vi "main(Test DQMH modules).vi"() -> ()   [LabVIEW 2018, in "Application.lvlib"] (continued)
                n6985 = To Variant(anything=bool[] [FALSE, FALSE, TRUE, FALSE, FALSE, FALSE]) -> (Variant=w14928:variant)
                n6986 = Bundle By Name(cluster=w14931, "command"="MEAS.AllRelaysOFF") -> (w14927:T9)
                n6987 = Bundle By Name(cluster=w14931, "command"="MEAS.mux10-1", "data"=w14938) -> (w14926:T9)
                n6988 = Bundle By Name(cluster=w14931, "command"="MEAS.mux6_1", "data"=w14936) -> (w14925:T9)
                n6989 = Bundle By Name(cluster=w14931, "command"="MEAS.demux1-10", "data"=w14932) -> (w14924:T9)
                n6990 = Bundle By Name(cluster=w14931, "command"="MEAS.eMIC", "data"=w14928) -> (w14923:T9)
                n6991 = Build Array(w14927, w14926, w14925, w14924, w14923) -> (w14908:T9[])
                n6992 = To Variant(anything=w14913) -> (Variant=w14911:variant)
                n6993 = To Variant(anything=w14913) -> (Variant=w14910:variant)
                n6994 = Bundle By Name(cluster=w14909, "command"="WaitFor") -> (w14907:T9)
                n6995 = Bundle By Name(cluster=w14909, "command"="MEAS.DMM dual read") -> (w14920:T9)
                n6996 = Bundle By Name(cluster=w14909, "command"="MEAS.requestAC", "data"=w14911) -> (w14919:T9)
                n6997 = Bundle By Name(cluster=w14909, "command"="Apps.WaitForEvent", "data"=w14910) -> (w14914:T9)
                n6998 = Bundle By Name(cluster=w14909, "command"="Apps.UI Update 1") -> (w14915:T9)
                n6999 = Build Array (concatenate)(w14908, w14907, w14920, w14919, w14914, w14915) -> (w14912:T9[])
              }
            }
          }
          frame True {
            n7000 = Bundle By Name(cluster=T9 {"command"="", "data"=variant} ("element"), "command"="Apps.UI Update 1") -> (w14942:T9)
            n7001 = Build Array(w14942) -> (w14941:T9[])
          }
        }
        n7002 = for {
          tunnel: w14857 -> [w14952] mode=indexing
          tunnel: w14865 -> [w14953]
          tunnel: [w14949] -> w14867 mode=indexing
          n7003 = Unbundle By Name(w14952) -> ("command"=w14951:string, "data"=w14950:variant)
          n7004 = call "App enquece.vi"("command data"=w14950, "command"=w14951, "queue in"=w14953) -> ("error out"=w14949:errorcluster)  [unwired: 7 in, 1 out]
        }
        n7005 = Merge Errors(w14868, w14867) -> (w14866:errorcluster)
      }
      frame "Test DRV 52A" {
        w14957 = 52 ("DUT index(0-59)")
        n7006 = disable-structure shown="LOGGING==TRUE" {
          disable-tunnel: w14962 -> [w15045 _]
          frame condition #0 (active) {
            n7007 = Empty String/Path?(string/path=w15045) -> (empty?=w15047:bool)
            n7008 = Select(t="Quece timeout", s=w15047, f=w15045) -> (s? t:f=w15044:string)
            n7009 = call "string log (SubVI).vi"("state Name"=w15044) -> ()  [unwired: 9 in, 2 out]
          }
          frame condition #1 {
          }
        }
        n7010 = Flush Queue(queue=w14963) -> (queue out=w14964:refnum<queue>)  [unwired: 1 in, 2 out]
        n7011 = Decrement(x=w14957) -> (x-1=w14961:i32)
        n7012 = Index Array(array=w14958, index=w14961) -> (element=w14959:refnum<vi>)
        n7013 = call "FGV DRV stand.vi"() -> ("Sub-Test.DCV"=w14954:bool)  [unwired: 10 in, 1 out]
        n7014 = call "FGV Driver Data.vi"("DUT index(1-60)"=w14957) -> ("DUT SC"=w14955:bool)  [unwired: 7 in, 3 out]
        n7015 = property class="ColBox"(reference=w14959, "Value"=u32 10000536 ("DRV 1")) -> ()  [unwired: 1 in, 2 out]
        n7016 = case shown="False" w14955 {
          tunnel: w14957 -> [w14975 _]
          tunnel: [w14974 w15040] -> w14956
          tunnel: w14954 -> [w14973 _]
          frame False {
            n7017 = case shown="False" w14973 {
              tunnel: w14975 -> [w14982 w15012]
              tunnel: [w14993 w15011] -> w14974
              frame False {
                w14979 = T9 {"command"="", "data"=variant} ("element")
                w14992 = T9 {"command"="", "data"=variant} ("element")
                n7018 = To Variant(anything=T3."mux10_1_channel9" ("mux10_1(x6)_encode")) -> (Variant=w14990:variant)
                n7019 = To Variant(anything=T4."demux1_10_channel9" ("demux1_10(x6)_encode")) -> (Variant=w14986:variant)
                n7020 = To Variant(anything=bool[] [FALSE, FALSE, FALSE, TRUE, FALSE, FALSE]) -> (Variant=w15001:variant)
                n7021 = Bundle By Name(cluster=w14992, "command"="MEAS.AllRelaysOFF") -> (w15000:T9)
                n7022 = Bundle By Name(cluster=w14992, "command"="MEAS.mux10-1", "data"=w14990) -> (w14983:T9)
                n7023 = Bundle By Name(cluster=w14992, "command"="MEAS.demux1-10", "data"=w14986) -> (w14984:T9)
                n7024 = Bundle By Name(cluster=w14992, "command"="MEAS.eMIC", "data"=w15001) -> (w14985:T9)
                n7025 = Build Array(w15000, w14983, w14984, w14985) -> (w14978:T9[])
                n7026 = To Variant(anything=w14982) -> (Variant=w14981:variant)
                n7027 = To Variant(anything=w14982) -> (Variant=w14980:variant)
                n7028 = Bundle By Name(cluster=w14979, "command"="MEAS.requestAC", "data"=w14981) -> (w14998:T9)
                n7029 = Bundle By Name(cluster=w14979, "command"="Apps.WaitForEvent", "data"=w14980) -> (w14994:T9)
                n7030 = Bundle By Name(cluster=w14979, "command"="Apps.UI Update 1") -> (w14995:T9)
                n7031 = Bundle By Name(cluster=w14979, "command"="WaitFor") -> (w14977:T9)
                n7032 = Build Array (concatenate)(w14978, w14977, w14998, w14994, w14995) -> (w14993:T9[])
              }
              frame True {
                w15008 = T9 {"command"="", "data"=variant} ("element")
                w15030 = T9 {"command"="", "data"=variant} ("element")
                n7033 = To Variant(anything=T3."mux10_1_channel9" ("mux10_1(x6)_encode")) -> (Variant=w15037:variant)
                n7034 = To Variant(anything=T2."mux6_1_channel4_3" ("mux6_1(3wires)_encode")) -> (Variant=w15035:variant)
                n7035 = To Variant(anything=T4."demux1_10_channel9" ("demux1_10(x6)_encode")) -> (Variant=w15031:variant)
                n7036 = To Variant(anything=bool[] [FALSE, FALSE, FALSE, TRUE, FALSE, FALSE]) -> (Variant=w15027:variant)
                n7037 = Bundle By Name(cluster=w15030, "command"="MEAS.AllRelaysOFF") -> (w15026:T9)
                n7038 = Bundle By Name(cluster=w15030, "command"="MEAS.mux10-1", "data"=w15037) -> (w15025:T9)
                n7039 = Bundle By Name(cluster=w15030, "command"="MEAS.mux6_1", "data"=w15035) -> (w15024:T9)
                n7040 = Bundle By Name(cluster=w15030, "command"="MEAS.demux1-10", "data"=w15031) -> (w15023:T9)
                n7041 = Bundle By Name(cluster=w15030, "command"="MEAS.eMIC", "data"=w15027) -> (w15022:T9)
                n7042 = Build Array(w15026, w15025, w15024, w15023, w15022) -> (w15007:T9[])
                n7043 = To Variant(anything=w15012) -> (Variant=w15010:variant)
                n7044 = To Variant(anything=w15012) -> (Variant=w15009:variant)
                n7045 = Bundle By Name(cluster=w15008, "command"="WaitFor") -> (w15006:T9)
                n7046 = Bundle By Name(cluster=w15008, "command"="MEAS.DMM dual read") -> (w15019:T9)
                n7047 = Bundle By Name(cluster=w15008, "command"="MEAS.requestAC", "data"=w15010) -> (w15018:T9)
                n7048 = Bundle By Name(cluster=w15008, "command"="Apps.WaitForEvent", "data"=w15009) -> (w15013:T9)
                n7049 = Bundle By Name(cluster=w15008, "command"="Apps.UI Update 1") -> (w15014:T9)
                n7050 = Build Array (concatenate)(w15007, w15006, w15019, w15018, w15013, w15014) -> (w15011:T9[])
              }
            }
          }
          frame True {
            n7051 = Bundle By Name(cluster=T9 {"command"="", "data"=variant} ("element"), "command"="Apps.UI Update 1") -> (w15041:T9)
            n7052 = Build Array(w15041) -> (w15040:T9[])
          }
        }
        n7053 = for {
          tunnel: w14956 -> [w15051] mode=indexing
          tunnel: w14964 -> [w15052]
          tunnel: [w15048] -> w14966 mode=indexing
          n7054 = Unbundle By Name(w15051) -> ("command"=w15050:string, "data"=w15049:variant)
          n7055 = call "App enquece.vi"("command data"=w15049, "command"=w15050, "queue in"=w15052) -> ("error out"=w15048:errorcluster)  [unwired: 7 in, 1 out]
        }
        n7056 = Merge Errors(w14967, w14966) -> (w14965:errorcluster)
      }
      frame "Test DRV 53A" {
        w15056 = 53 ("DUT index(0-59)")
        n7057 = disable-structure shown="LOGGING==TRUE" {
          disable-tunnel: w15061 -> [w15144 _]
          frame condition #0 (active) {
            n7058 = Empty String/Path?(string/path=w15144) -> (empty?=w15146:bool)
            n7059 = Select(t="Quece timeout", s=w15146, f=w15144) -> (s? t:f=w15143:string)
            n7060 = call "string log (SubVI).vi"("state Name"=w15143) -> ()  [unwired: 9 in, 2 out]
          }
          frame condition #1 {
          }
        }
        n7061 = Flush Queue(queue=w15062) -> (queue out=w15063:refnum<queue>)  [unwired: 1 in, 2 out]
        n7062 = Decrement(x=w15056) -> (x-1=w15060:i32)
        n7063 = Index Array(array=w15057, index=w15060) -> (element=w15058:refnum<vi>)
        n7064 = call "FGV DRV stand.vi"() -> ("Sub-Test.DCV"=w15053:bool)  [unwired: 10 in, 1 out]
        n7065 = call "FGV Driver Data.vi"("DUT index(1-60)"=w15056) -> ("DUT SC"=w15054:bool)  [unwired: 7 in, 3 out]
        n7066 = property class="ColBox"(reference=w15058, "Value"=u32 10000536 ("DRV 1")) -> ()  [unwired: 1 in, 2 out]
        n7067 = case shown="False" w15054 {
          tunnel: w15056 -> [w15074 _]
          tunnel: [w15073 w15139] -> w15055
          tunnel: w15053 -> [w15072 _]
          frame False {
            n7068 = case shown="True" w15072 {
              tunnel: w15074 -> [w15081 w15111]
              tunnel: [w15092 w15110] -> w15073
              frame False {
                w15078 = T9 {"command"="", "data"=variant} ("element")
                w15091 = T9 {"command"="", "data"=variant} ("element")
                n7069 = To Variant(anything=T3."mux10_1_channel9" ("mux10_1(x6)_encode")) -> (Variant=w15089:variant)
                n7070 = To Variant(anything=T4."demux1_10_channel9" ("demux1_10(x6)_encode")) -> (Variant=w15085:variant)
                n7071 = To Variant(anything=bool[] [FALSE, FALSE, FALSE, FALSE, TRUE, FALSE]) -> (Variant=w15100:variant)
                n7072 = Bundle By Name(cluster=w15091, "command"="MEAS.AllRelaysOFF") -> (w15099:T9)
                n7073 = Bundle By Name(cluster=w15091, "command"="MEAS.mux10-1", "data"=w15089) -> (w15082:T9)
                n7074 = Bundle By Name(cluster=w15091, "command"="MEAS.demux1-10", "data"=w15085) -> (w15083:T9)
                n7075 = Bundle By Name(cluster=w15091, "command"="MEAS.eMIC", "data"=w15100) -> (w15084:T9)
                n7076 = Build Array(w15099, w15082, w15083, w15084) -> (w15077:T9[])
                n7077 = To Variant(anything=w15081) -> (Variant=w15080:variant)
                n7078 = To Variant(anything=w15081) -> (Variant=w15079:variant)
                n7079 = Bundle By Name(cluster=w15078, "command"="MEAS.requestAC", "data"=w15080) -> (w15097:T9)
                n7080 = Bundle By Name(cluster=w15078, "command"="Apps.WaitForEvent", "data"=w15079) -> (w15093:T9)
                n7081 = Bundle By Name(cluster=w15078, "command"="Apps.UI Update 1") -> (w15094:T9)
                n7082 = Bundle By Name(cluster=w15078, "command"="WaitFor") -> (w15076:T9)
                n7083 = Build Array (concatenate)(w15077, w15076, w15097, w15093, w15094) -> (w15092:T9[])
              }
              frame True {
                w15107 = T9 {"command"="", "data"=variant} ("element")
                w15129 = T9 {"command"="", "data"=variant} ("element")
                n7084 = To Variant(anything=T3."mux10_1_channel9" ("mux10_1(x6)_encode")) -> (Variant=w15136:variant)
                n7085 = To Variant(anything=T2."mux6_1_channel5_3" ("mux6_1(3wires)_encode")) -> (Variant=w15134:variant)
                n7086 = To Variant(anything=T4."demux1_10_channel9" ("demux1_10(x6)_encode")) -> (Variant=w15130:variant)
                n7087 = To Variant(anything=bool[] [FALSE, FALSE, FALSE, FALSE, TRUE, FALSE]) -> (Variant=w15126:variant)
                n7088 = Bundle By Name(cluster=w15129, "command"="MEAS.AllRelaysOFF") -> (w15125:T9)
                n7089 = Bundle By Name(cluster=w15129, "command"="MEAS.mux10-1", "data"=w15136) -> (w15124:T9)
                n7090 = Bundle By Name(cluster=w15129, "command"="MEAS.mux6_1", "data"=w15134) -> (w15123:T9)
                n7091 = Bundle By Name(cluster=w15129, "command"="MEAS.demux1-10", "data"=w15130) -> (w15122:T9)
                n7092 = Bundle By Name(cluster=w15129, "command"="MEAS.eMIC", "data"=w15126) -> (w15121:T9)
                n7093 = Build Array(w15125, w15124, w15123, w15122, w15121) -> (w15106:T9[])
                n7094 = To Variant(anything=w15111) -> (Variant=w15109:variant)
                n7095 = To Variant(anything=w15111) -> (Variant=w15108:variant)
                n7096 = Bundle By Name(cluster=w15107, "command"="WaitFor") -> (w15105:T9)
                n7097 = Bundle By Name(cluster=w15107, "command"="MEAS.DMM dual read") -> (w15118:T9)
                n7098 = Bundle By Name(cluster=w15107, "command"="MEAS.requestAC", "data"=w15109) -> (w15117:T9)
                n7099 = Bundle By Name(cluster=w15107, "command"="Apps.WaitForEvent", "data"=w15108) -> (w15112:T9)
                n7100 = Bundle By Name(cluster=w15107, "command"="Apps.UI Update 1") -> (w15113:T9)
                n7101 = Build Array (concatenate)(w15106, w15105, w15118, w15117, w15112, w15113) -> (w15110:T9[])
              }
            }
          }
          frame True {
            n7102 = Bundle By Name(cluster=T9 {"command"="", "data"=variant} ("element"), "command"="Apps.UI Update 1") -> (w15140:T9)
            n7103 = Build Array(w15140) -> (w15139:T9[])
          }
        }
        n7104 = for {
          tunnel: w15055 -> [w15150] mode=indexing
          tunnel: w15063 -> [w15151]
          tunnel: [w15147] -> w15065 mode=indexing
          n7105 = Unbundle By Name(w15150) -> ("command"=w15149:string, "data"=w15148:variant)
          n7106 = call "App enquece.vi"("command data"=w15148, "command"=w15149, "queue in"=w15151) -> ("error out"=w15147:errorcluster)  [unwired: 7 in, 1 out]
        }
        n7107 = Merge Errors(w15066, w15065) -> (w15064:errorcluster)
      }
      frame "Test DRV 54A" {
        w15155 = 54 ("DUT index(0-59)")
        n7108 = disable-structure shown="LOGGING==TRUE" {
          disable-tunnel: w15160 -> [w15243 _]
          frame condition #0 (active) {
            n7109 = Empty String/Path?(string/path=w15243) -> (empty?=w15245:bool)
            n7110 = Select(t="Quece timeout", s=w15245, f=w15243) -> (s? t:f=w15242:string)
            n7111 = call "string log (SubVI).vi"("state Name"=w15242) -> ()  [unwired: 9 in, 2 out]
          }
          frame condition #1 {
          }
        }
        n7112 = Flush Queue(queue=w15161) -> (queue out=w15162:refnum<queue>)  [unwired: 1 in, 2 out]
        n7113 = Decrement(x=w15155) -> (x-1=w15159:i32)
        n7114 = Index Array(array=w15156, index=w15159) -> (element=w15157:refnum<vi>)
        n7115 = call "FGV DRV stand.vi"() -> ("Sub-Test.DCV"=w15152:bool)  [unwired: 10 in, 1 out]
        n7116 = call "FGV Driver Data.vi"("DUT index(1-60)"=w15155) -> ("DUT SC"=w15153:bool)  [unwired: 7 in, 3 out]
        n7117 = property class="ColBox"(reference=w15157, "Value"=u32 10000536 ("DRV 1")) -> ()  [unwired: 1 in, 2 out]
        n7118 = case shown="False" w15153 {
          tunnel: w15155 -> [w15173 _]
          tunnel: [w15172 w15238] -> w15154
          tunnel: w15152 -> [w15171 _]
          frame False {
            n7119 = case shown="False" w15171 {
              tunnel: w15173 -> [w15180 w15210]
              tunnel: [w15191 w15209] -> w15172
              frame False {
                w15177 = T9 {"command"="", "data"=variant} ("element")
                w15190 = T9 {"command"="", "data"=variant} ("element")
                n7120 = To Variant(anything=T3."mux10_1_channel9" ("mux10_1(x6)_encode")) -> (Variant=w15188:variant)
                n7121 = To Variant(anything=T4."demux1_10_channel9" ("demux1_10(x6)_encode")) -> (Variant=w15184:variant)
                n7122 = To Variant(anything=bool[] [FALSE, FALSE, FALSE, FALSE, FALSE, TRUE]) -> (Variant=w15199:variant)
                n7123 = Bundle By Name(cluster=w15190, "command"="MEAS.AllRelaysOFF") -> (w15198:T9)
                n7124 = Bundle By Name(cluster=w15190, "command"="MEAS.mux10-1", "data"=w15188) -> (w15181:T9)
                n7125 = Bundle By Name(cluster=w15190, "command"="MEAS.demux1-10", "data"=w15184) -> (w15182:T9)
                n7126 = Bundle By Name(cluster=w15190, "command"="MEAS.eMIC", "data"=w15199) -> (w15183:T9)
                n7127 = Build Array(w15198, w15181, w15182, w15183) -> (w15176:T9[])
                n7128 = To Variant(anything=w15180) -> (Variant=w15179:variant)
                n7129 = To Variant(anything=w15180) -> (Variant=w15178:variant)
                n7130 = Bundle By Name(cluster=w15177, "command"="MEAS.requestAC", "data"=w15179) -> (w15196:T9)
                n7131 = Bundle By Name(cluster=w15177, "command"="Apps.WaitForEvent", "data"=w15178) -> (w15192:T9)
                n7132 = Bundle By Name(cluster=w15177, "command"="Apps.UI Update 1") -> (w15193:T9)
                n7133 = Bundle By Name(cluster=w15177, "command"="WaitFor") -> (w15175:T9)
                n7134 = Build Array (concatenate)(w15176, w15175, w15196, w15192, w15193) -> (w15191:T9[])
              }
              frame True {
                w15206 = T9 {"command"="", "data"=variant} ("element")
                w15228 = T9 {"command"="", "data"=variant} ("element")
                n7135 = To Variant(anything=T3."mux10_1_channel9" ("mux10_1(x6)_encode")) -> (Variant=w15235:variant)
                n7136 = To Variant(anything=T2."mux6_1_channel6_3" ("mux6_1(3wires)_encode")) -> (Variant=w15233:variant)
                n7137 = To Variant(anything=T4."demux1_10_channel9" ("demux1_10(x6)_encode")) -> (Variant=w15229:variant)
                n7138 = To Variant(anything=bool[] [FALSE, FALSE, FALSE, FALSE, FALSE, TRUE]) -> (Variant=w15225:variant)
                n7139 = Bundle By Name(cluster=w15228, "command"="MEAS.AllRelaysOFF") -> (w15224:T9)
                n7140 = Bundle By Name(cluster=w15228, "command"="MEAS.mux10-1", "data"=w15235) -> (w15223:T9)
                n7141 = Bundle By Name(cluster=w15228, "command"="MEAS.mux6_1", "data"=w15233) -> (w15222:T9)
                n7142 = Bundle By Name(cluster=w15228, "command"="MEAS.demux1-10", "data"=w15229) -> (w15221:T9)
                n7143 = Bundle By Name(cluster=w15228, "command"="MEAS.eMIC", "data"=w15225) -> (w15220:T9)
                n7144 = Build Array(w15224, w15223, w15222, w15221, w15220) -> (w15205:T9[])
                n7145 = To Variant(anything=w15210) -> (Variant=w15208:variant)
                n7146 = To Variant(anything=w15210) -> (Variant=w15207:variant)
                n7147 = Bundle By Name(cluster=w15206, "command"="WaitFor") -> (w15204:T9)
                n7148 = Bundle By Name(cluster=w15206, "command"="MEAS.DMM dual read") -> (w15217:T9)
                n7149 = Bundle By Name(cluster=w15206, "command"="MEAS.requestAC", "data"=w15208) -> (w15216:T9)
                n7150 = Bundle By Name(cluster=w15206, "command"="Apps.WaitForEvent", "data"=w15207) -> (w15211:T9)
                n7151 = Bundle By Name(cluster=w15206, "command"="Apps.UI Update 1") -> (w15212:T9)
                n7152 = Build Array (concatenate)(w15205, w15204, w15217, w15216, w15211, w15212) -> (w15209:T9[])
              }
            }
          }
          frame True {
            n7153 = Bundle By Name(cluster=T9 {"command"="", "data"=variant} ("element"), "command"="Apps.UI Update 1") -> (w15239:T9)
            n7154 = Build Array(w15239) -> (w15238:T9[])
          }
        }
        n7155 = for {
          tunnel: w15154 -> [w15249] mode=indexing
          tunnel: w15162 -> [w15250]
          tunnel: [w15246] -> w15164 mode=indexing
          n7156 = Unbundle By Name(w15249) -> ("command"=w15248:string, "data"=w15247:variant)
          n7157 = call "App enquece.vi"("command data"=w15247, "command"=w15248, "queue in"=w15250) -> ("error out"=w15246:errorcluster)  [unwired: 7 in, 1 out]
        }
        n7158 = Merge Errors(w15165, w15164) -> (w15163:errorcluster)
      }
      frame "Test DRV 55A" {
        w15254 = 55 ("DUT index(0-59)")
        n7159 = disable-structure shown="LOGGING==TRUE" {
          disable-tunnel: w15259 -> [w15342 _]
          frame condition #0 (active) {
            n7160 = Empty String/Path?(string/path=w15342) -> (empty?=w15344:bool)
            n7161 = Select(t="Quece timeout", s=w15344, f=w15342) -> (s? t:f=w15341:string)
            n7162 = call "string log (SubVI).vi"("state Name"=w15341) -> ()  [unwired: 9 in, 2 out]
          }
          frame condition #1 {
          }
        }
        n7163 = Flush Queue(queue=w15260) -> (queue out=w15261:refnum<queue>)  [unwired: 1 in, 2 out]
        n7164 = Decrement(x=w15254) -> (x-1=w15258:i32)
        n7165 = Index Array(array=w15255, index=w15258) -> (element=w15256:refnum<vi>)
        n7166 = call "FGV DRV stand.vi"() -> ("Sub-Test.DCV"=w15251:bool)  [unwired: 10 in, 1 out]
        n7167 = call "FGV Driver Data.vi"("DUT index(1-60)"=w15254) -> ("DUT SC"=w15252:bool)  [unwired: 7 in, 3 out]
        n7168 = property class="ColBox"(reference=w15256, "Value"=u32 10000536 ("DRV 1")) -> ()  [unwired: 1 in, 2 out]
        n7169 = case shown="False" w15252 {
          tunnel: w15254 -> [w15272 _]
          tunnel: [w15271 w15337] -> w15253
          tunnel: w15251 -> [w15270 _]
          frame False {
            n7170 = case shown="True" w15270 {
              tunnel: w15272 -> [w15279 w15309]
              tunnel: [w15290 w15308] -> w15271
              frame False {
                w15276 = T9 {"command"="", "data"=variant} ("element")
                w15289 = T9 {"command"="", "data"=variant} ("element")
                n7171 = To Variant(anything=T3."mux10_1_channel10" ("mux10_1(x6)_encode")) -> (Variant=w15287:variant)
                n7172 = To Variant(anything=T4."demux1_10_channel10" ("demux1_10(x6)_encode")) -> (Variant=w15283:variant)
                n7173 = To Variant(anything=bool[] [TRUE, FALSE, FALSE, FALSE, FALSE, FALSE]) -> (Variant=w15298:variant)
                n7174 = Bundle By Name(cluster=w15289, "command"="MEAS.AllRelaysOFF") -> (w15297:T9)
                n7175 = Bundle By Name(cluster=w15289, "command"="MEAS.mux10-1", "data"=w15287) -> (w15280:T9)
                n7176 = Bundle By Name(cluster=w15289, "command"="MEAS.demux1-10", "data"=w15283) -> (w15281:T9)
                n7177 = Bundle By Name(cluster=w15289, "command"="MEAS.eMIC", "data"=w15298) -> (w15282:T9)
                n7178 = Build Array(w15297, w15280, w15281, w15282) -> (w15275:T9[])
                n7179 = To Variant(anything=w15279) -> (Variant=w15278:variant)
                n7180 = To Variant(anything=w15279) -> (Variant=w15277:variant)
                n7181 = Bundle By Name(cluster=w15276, "command"="MEAS.requestAC", "data"=w15278) -> (w15295:T9)
                n7182 = Bundle By Name(cluster=w15276, "command"="Apps.WaitForEvent", "data"=w15277) -> (w15291:T9)
                n7183 = Bundle By Name(cluster=w15276, "command"="Apps.UI Update 1") -> (w15292:T9)
                n7184 = Bundle By Name(cluster=w15276, "command"="WaitFor") -> (w15274:T9)
                n7185 = Build Array (concatenate)(w15275, w15274, w15295, w15291, w15292) -> (w15290:T9[])
              }
              frame True {
                w15305 = T9 {"command"="", "data"=variant} ("element")
                w15327 = T9 {"command"="", "data"=variant} ("element")
                n7186 = To Variant(anything=T3."mux10_1_channel10" ("mux10_1(x6)_encode")) -> (Variant=w15334:variant)
                n7187 = To Variant(anything=T2."mux6_1_channel1_3" ("mux6_1(3wires)_encode")) -> (Variant=w15332:variant)
                n7188 = To Variant(anything=T4."demux1_10_channel10" ("demux1_10(x6)_encode")) -> (Variant=w15328:variant)
                n7189 = To Variant(anything=bool[] [TRUE, FALSE, FALSE, FALSE, FALSE, FALSE]) -> (Variant=w15324:variant)
                n7190 = Bundle By Name(cluster=w15327, "command"="MEAS.AllRelaysOFF") -> (w15323:T9)
                n7191 = Bundle By Name(cluster=w15327, "command"="MEAS.mux10-1", "data"=w15334) -> (w15322:T9)
                n7192 = Bundle By Name(cluster=w15327, "command"="MEAS.mux6_1", "data"=w15332) -> (w15321:T9)
                n7193 = Bundle By Name(cluster=w15327, "command"="MEAS.demux1-10", "data"=w15328) -> (w15320:T9)
                n7194 = Bundle By Name(cluster=w15327, "command"="MEAS.eMIC", "data"=w15324) -> (w15319:T9)
                n7195 = Build Array(w15323, w15322, w15321, w15320, w15319) -> (w15304:T9[])
                n7196 = To Variant(anything=w15309) -> (Variant=w15307:variant)
                n7197 = To Variant(anything=w15309) -> (Variant=w15306:variant)
                n7198 = Bundle By Name(cluster=w15305, "command"="WaitFor") -> (w15303:T9)
                n7199 = Bundle By Name(cluster=w15305, "command"="MEAS.DMM dual read") -> (w15316:T9)
                n7200 = Bundle By Name(cluster=w15305, "command"="MEAS.requestAC", "data"=w15307) -> (w15315:T9)
                n7201 = Bundle By Name(cluster=w15305, "command"="Apps.WaitForEvent", "data"=w15306) -> (w15310:T9)
                n7202 = Bundle By Name(cluster=w15305, "command"="Apps.UI Update 1") -> (w15311:T9)
                n7203 = Build Array (concatenate)(w15304, w15303, w15316, w15315, w15310, w15311) -> (w15308:T9[])
              }
            }
          }
          frame True {
            n7204 = Bundle By Name(cluster=T9 {"command"="", "data"=variant} ("element"), "command"="Apps.UI Update 1") -> (w15338:T9)
            n7205 = Build Array(w15338) -> (w15337:T9[])
          }
        }
        n7206 = for {
          tunnel: w15253 -> [w15348] mode=indexing
          tunnel: w15261 -> [w15349]
          tunnel: [w15345] -> w15263 mode=indexing
          n7207 = Unbundle By Name(w15348) -> ("command"=w15347:string, "data"=w15346:variant)
          n7208 = call "App enquece.vi"("command data"=w15346, "command"=w15347, "queue in"=w15349) -> ("error out"=w15345:errorcluster)  [unwired: 7 in, 1 out]
        }
        n7209 = Merge Errors(w15264, w15263) -> (w15262:errorcluster)
      }
      frame "Test DRV 56A" {
        w15353 = 56 ("DUT index(0-59)")
        n7210 = disable-structure shown="LOGGING==TRUE" {
          disable-tunnel: w15358 -> [w15441 _]
          frame condition #0 (active) {
            n7211 = Empty String/Path?(string/path=w15441) -> (empty?=w15443:bool)
            n7212 = Select(t="Quece timeout", s=w15443, f=w15441) -> (s? t:f=w15440:string)
            n7213 = call "string log (SubVI).vi"("state Name"=w15440) -> ()  [unwired: 9 in, 2 out]
          }
          frame condition #1 {
          }
        }
        n7214 = Flush Queue(queue=w15359) -> (queue out=w15360:refnum<queue>)  [unwired: 1 in, 2 out]
        n7215 = Decrement(x=w15353) -> (x-1=w15357:i32)
        n7216 = Index Array(array=w15354, index=w15357) -> (element=w15355:refnum<vi>)
        n7217 = call "FGV DRV stand.vi"() -> ("Sub-Test.DCV"=w15350:bool)  [unwired: 10 in, 1 out]
        n7218 = call "FGV Driver Data.vi"("DUT index(1-60)"=w15353) -> ("DUT SC"=w15351:bool)  [unwired: 7 in, 3 out]
        n7219 = property class="ColBox"(reference=w15355, "Value"=u32 10000536 ("DRV 1")) -> ()  [unwired: 1 in, 2 out]
        n7220 = case shown="False" w15351 {
          tunnel: w15353 -> [w15371 _]
          tunnel: [w15370 w15436] -> w15352
          tunnel: w15350 -> [w15369 _]
          frame False {
            n7221 = case shown="False" w15369 {
              tunnel: w15371 -> [w15378 w15408]
              tunnel: [w15389 w15407] -> w15370
              frame False {
                w15375 = T9 {"command"="", "data"=variant} ("element")
                w15388 = T9 {"command"="", "data"=variant} ("element")
                n7222 = To Variant(anything=T3."mux10_1_channel10" ("mux10_1(x6)_encode")) -> (Variant=w15386:variant)
                n7223 = To Variant(anything=T4."demux1_10_channel10" ("demux1_10(x6)_encode")) -> (Variant=w15382:variant)
                n7224 = To Variant(anything=bool[] [FALSE, TRUE, FALSE, FALSE, FALSE, FALSE]) -> (Variant=w15397:variant)
                n7225 = Bundle By Name(cluster=w15388, "command"="MEAS.AllRelaysOFF") -> (w15396:T9)
                n7226 = Bundle By Name(cluster=w15388, "command"="MEAS.mux10-1", "data"=w15386) -> (w15379:T9)
                n7227 = Bundle By Name(cluster=w15388, "command"="MEAS.demux1-10", "data"=w15382) -> (w15380:T9)
                n7228 = Bundle By Name(cluster=w15388, "command"="MEAS.eMIC", "data"=w15397) -> (w15381:T9)
                n7229 = Build Array(w15396, w15379, w15380, w15381) -> (w15374:T9[])
                n7230 = To Variant(anything=w15378) -> (Variant=w15377:variant)
                n7231 = To Variant(anything=w15378) -> (Variant=w15376:variant)
                n7232 = Bundle By Name(cluster=w15375, "command"="MEAS.requestAC", "data"=w15377) -> (w15394:T9)
                n7233 = Bundle By Name(cluster=w15375, "command"="Apps.WaitForEvent", "data"=w15376) -> (w15390:T9)
                n7234 = Bundle By Name(cluster=w15375, "command"="Apps.UI Update 1") -> (w15391:T9)
                n7235 = Bundle By Name(cluster=w15375, "command"="WaitFor") -> (w15373:T9)
                n7236 = Build Array (concatenate)(w15374, w15373, w15394, w15390, w15391) -> (w15389:T9[])
              }
              frame True {
                w15404 = T9 {"command"="", "data"=variant} ("element")
                w15426 = T9 {"command"="", "data"=variant} ("element")
                n7237 = To Variant(anything=T3."mux10_1_channel10" ("mux10_1(x6)_encode")) -> (Variant=w15433:variant)
                n7238 = To Variant(anything=T2."mux6_1_channel2_3" ("mux6_1(3wires)_encode")) -> (Variant=w15431:variant)
                n7239 = To Variant(anything=T4."demux1_10_channel10" ("demux1_10(x6)_encode")) -> (Variant=w15427:variant)
                n7240 = To Variant(anything=bool[] [FALSE, TRUE, FALSE, FALSE, FALSE, FALSE]) -> (Variant=w15423:variant)
                n7241 = Bundle By Name(cluster=w15426, "command"="MEAS.AllRelaysOFF") -> (w15422:T9)
                n7242 = Bundle By Name(cluster=w15426, "command"="MEAS.mux10-1", "data"=w15433) -> (w15421:T9)
                n7243 = Bundle By Name(cluster=w15426, "command"="MEAS.mux6_1", "data"=w15431) -> (w15420:T9)
                n7244 = Bundle By Name(cluster=w15426, "command"="MEAS.demux1-10", "data"=w15427) -> (w15419:T9)
                n7245 = Bundle By Name(cluster=w15426, "command"="MEAS.eMIC", "data"=w15423) -> (w15418:T9)
                n7246 = Build Array(w15422, w15421, w15420, w15419, w15418) -> (w15403:T9[])
                n7247 = To Variant(anything=w15408) -> (Variant=w15406:variant)
                n7248 = To Variant(anything=w15408) -> (Variant=w15405:variant)
                n7249 = Bundle By Name(cluster=w15404, "command"="WaitFor") -> (w15402:T9)
                n7250 = Bundle By Name(cluster=w15404, "command"="MEAS.DMM dual read") -> (w15415:T9)
                n7251 = Bundle By Name(cluster=w15404, "command"="MEAS.requestAC", "data"=w15406) -> (w15414:T9)
                n7252 = Bundle By Name(cluster=w15404, "command"="Apps.WaitForEvent", "data"=w15405) -> (w15409:T9)
                n7253 = Bundle By Name(cluster=w15404, "command"="Apps.UI Update 1") -> (w15410:T9)
                n7254 = Build Array (concatenate)(w15403, w15402, w15415, w15414, w15409, w15410) -> (w15407:T9[])
              }
            }
          }
          frame True {
            n7255 = Bundle By Name(cluster=T9 {"command"="", "data"=variant} ("element"), "command"="Apps.UI Update 1") -> (w15437:T9)
            n7256 = Build Array(w15437) -> (w15436:T9[])
          }
        }
        n7257 = for {
          tunnel: w15352 -> [w15447] mode=indexing
          tunnel: w15360 -> [w15448]
          tunnel: [w15444] -> w15362 mode=indexing
          n7258 = Unbundle By Name(w15447) -> ("command"=w15446:string, "data"=w15445:variant)
          n7259 = call "App enquece.vi"("command data"=w15445, "command"=w15446, "queue in"=w15448) -> ("error out"=w15444:errorcluster)  [unwired: 7 in, 1 out]
        }
        n7260 = Merge Errors(w15363, w15362) -> (w15361:errorcluster)
      }
      frame "Test DRV 57A" {
        w15452 = 57 ("DUT index(0-59)")
        n7261 = disable-structure shown="LOGGING==TRUE" {
          disable-tunnel: w15457 -> [w15540 _]
          frame condition #0 (active) {
            n7262 = Empty String/Path?(string/path=w15540) -> (empty?=w15542:bool)
            n7263 = Select(t="Quece timeout", s=w15542, f=w15540) -> (s? t:f=w15539:string)
            n7264 = call "string log (SubVI).vi"("state Name"=w15539) -> ()  [unwired: 9 in, 2 out]
          }
          frame condition #1 {
          }
        }
        n7265 = Flush Queue(queue=w15458) -> (queue out=w15459:refnum<queue>)  [unwired: 1 in, 2 out]
        n7266 = Decrement(x=w15452) -> (x-1=w15456:i32)
        n7267 = Index Array(array=w15453, index=w15456) -> (element=w15454:refnum<vi>)
        n7268 = call "FGV DRV stand.vi"() -> ("Sub-Test.DCV"=w15449:bool)  [unwired: 10 in, 1 out]
        n7269 = call "FGV Driver Data.vi"("DUT index(1-60)"=w15452) -> ("DUT SC"=w15450:bool)  [unwired: 7 in, 3 out]
        n7270 = property class="ColBox"(reference=w15454, "Value"=u32 10000536 ("DRV 1")) -> ()  [unwired: 1 in, 2 out]
        n7271 = case shown="False" w15450 {
          tunnel: w15452 -> [w15470 _]
          tunnel: [w15469 w15535] -> w15451
          tunnel: w15449 -> [w15468 _]
          frame False {
            n7272 = case shown="True" w15468 {
              tunnel: w15470 -> [w15477 w15507]
              tunnel: [w15488 w15506] -> w15469
              frame False {
                w15474 = T9 {"command"="", "data"=variant} ("element")
                w15487 = T9 {"command"="", "data"=variant} ("element")
                n7273 = To Variant(anything=T3."mux10_1_channel10" ("mux10_1(x6)_encode")) -> (Variant=w15485:variant)
                n7274 = To Variant(anything=T4."demux1_10_channel10" ("demux1_10(x6)_encode")) -> (Variant=w15481:variant)
                n7275 = To Variant(anything=bool[] [FALSE, FALSE, TRUE, FALSE, FALSE, FALSE]) -> (Variant=w15496:variant)
                n7276 = Bundle By Name(cluster=w15487, "command"="MEAS.AllRelaysOFF") -> (w15495:T9)
                n7277 = Bundle By Name(cluster=w15487, "command"="MEAS.mux10-1", "data"=w15485) -> (w15478:T9)
                n7278 = Bundle By Name(cluster=w15487, "command"="MEAS.demux1-10", "data"=w15481) -> (w15479:T9)
                n7279 = Bundle By Name(cluster=w15487, "command"="MEAS.eMIC", "data"=w15496) -> (w15480:T9)
                n7280 = Build Array(w15495, w15478, w15479, w15480) -> (w15473:T9[])
                n7281 = To Variant(anything=w15477) -> (Variant=w15476:variant)
                n7282 = To Variant(anything=w15477) -> (Variant=w15475:variant)
                n7283 = Bundle By Name(cluster=w15474, "command"="MEAS.requestAC", "data"=w15476) -> (w15493:T9)
                n7284 = Bundle By Name(cluster=w15474, "command"="Apps.WaitForEvent", "data"=w15475) -> (w15489:T9)
                n7285 = Bundle By Name(cluster=w15474, "command"="Apps.UI Update 1") -> (w15490:T9)
                n7286 = Bundle By Name(cluster=w15474, "command"="WaitFor") -> (w15472:T9)
                n7287 = Build Array (concatenate)(w15473, w15472, w15493, w15489, w15490) -> (w15488:T9[])
              }
              frame True {
                w15503 = T9 {"command"="", "data"=variant} ("element")
                w15525 = T9 {"command"="", "data"=variant} ("element")
                n7288 = To Variant(anything=T3."mux10_1_channel10" ("mux10_1(x6)_encode")) -> (Variant=w15532:variant)
                n7289 = To Variant(anything=T2."mux6_1_channel3_3" ("mux6_1(3wires)_encode")) -> (Variant=w15530:variant)
                n7290 = To Variant(anything=T4."demux1_10_channel10" ("demux1_10(x6)_encode")) -> (Variant=w15526:variant)
                n7291 = To Variant(anything=bool[] [FALSE, FALSE, TRUE, FALSE, FALSE, FALSE]) -> (Variant=w15522:variant)
                n7292 = Bundle By Name(cluster=w15525, "command"="MEAS.AllRelaysOFF") -> (w15521:T9)
                n7293 = Bundle By Name(cluster=w15525, "command"="MEAS.mux10-1", "data"=w15532) -> (w15520:T9)
                n7294 = Bundle By Name(cluster=w15525, "command"="MEAS.mux6_1", "data"=w15530) -> (w15519:T9)
                n7295 = Bundle By Name(cluster=w15525, "command"="MEAS.demux1-10", "data"=w15526) -> (w15518:T9)
                n7296 = Bundle By Name(cluster=w15525, "command"="MEAS.eMIC", "data"=w15522) -> (w15517:T9)
                n7297 = Build Array(w15521, w15520, w15519, w15518, w15517) -> (w15502:T9[])
                n7298 = To Variant(anything=w15507) -> (Variant=w15505:variant)
                n7299 = To Variant(anything=w15507) -> (Variant=w15504:variant)
                n7300 = Bundle By Name(cluster=w15503, "command"="WaitFor") -> (w15501:T9)
                n7301 = Bundle By Name(cluster=w15503, "command"="MEAS.DMM dual read") -> (w15514:T9)
                n7302 = Bundle By Name(cluster=w15503, "command"="MEAS.requestAC", "data"=w15505) -> (w15513:T9)
                n7303 = Bundle By Name(cluster=w15503, "command"="Apps.WaitForEvent", "data"=w15504) -> (w15508:T9)
                n7304 = Bundle By Name(cluster=w15503, "command"="Apps.UI Update 1") -> (w15509:T9)
                n7305 = Build Array (concatenate)(w15502, w15501, w15514, w15513, w15508, w15509) -> (w15506:T9[])
              }
            }
          }
          frame True {
            n7306 = Bundle By Name(cluster=T9 {"command"="", "data"=variant} ("element"), "command"="Apps.UI Update 1") -> (w15536:T9)
            n7307 = Build Array(w15536) -> (w15535:T9[])
          }
        }
        n7308 = for {
          tunnel: w15451 -> [w15546] mode=indexing
          tunnel: w15459 -> [w15547]
          tunnel: [w15543] -> w15461 mode=indexing
          n7309 = Unbundle By Name(w15546) -> ("command"=w15545:string, "data"=w15544:variant)
          n7310 = call "App enquece.vi"("command data"=w15544, "command"=w15545, "queue in"=w15547) -> ("error out"=w15543:errorcluster)  [unwired: 7 in, 1 out]
        }
        n7311 = Merge Errors(w15462, w15461) -> (w15460:errorcluster)
      }
      frame "Test DRV 58A" {
        w15551 = 58 ("DUT index(0-59)")
        n7312 = disable-structure shown="LOGGING==TRUE" {
          disable-tunnel: w15556 -> [w15639 _]
          frame condition #0 (active) {
            n7313 = Empty String/Path?(string/path=w15639) -> (empty?=w15641:bool)
            n7314 = Select(t="Quece timeout", s=w15641, f=w15639) -> (s? t:f=w15638:string)
            n7315 = call "string log (SubVI).vi"("state Name"=w15638) -> ()  [unwired: 9 in, 2 out]
          }
          frame condition #1 {
          }
        }
        n7316 = Flush Queue(queue=w15557) -> (queue out=w15558:refnum<queue>)  [unwired: 1 in, 2 out]
        n7317 = Decrement(x=w15551) -> (x-1=w15555:i32)
        n7318 = Index Array(array=w15552, index=w15555) -> (element=w15553:refnum<vi>)
        n7319 = call "FGV DRV stand.vi"() -> ("Sub-Test.DCV"=w15548:bool)  [unwired: 10 in, 1 out]
        n7320 = call "FGV Driver Data.vi"("DUT index(1-60)"=w15551) -> ("DUT SC"=w15549:bool)  [unwired: 7 in, 3 out]
        n7321 = property class="ColBox"(reference=w15553, "Value"=u32 10000536 ("DRV 1")) -> ()  [unwired: 1 in, 2 out]
        n7322 = case shown="False" w15549 {
          tunnel: w15551 -> [w15569 _]
          tunnel: [w15568 w15634] -> w15550
          tunnel: w15548 -> [w15567 _]
          frame False {
            n7323 = case shown="False" w15567 {
              tunnel: w15569 -> [w15576 w15606]
              tunnel: [w15587 w15605] -> w15568
              frame False {
                w15573 = T9 {"command"="", "data"=variant} ("element")
                w15586 = T9 {"command"="", "data"=variant} ("element")
                n7324 = To Variant(anything=T3."mux10_1_channel10" ("mux10_1(x6)_encode")) -> (Variant=w15584:variant)
                n7325 = To Variant(anything=T4."demux1_10_channel10" ("demux1_10(x6)_encode")) -> (Variant=w15580:variant)
                n7326 = To Variant(anything=bool[] [FALSE, FALSE, FALSE, TRUE, FALSE, FALSE]) -> (Variant=w15595:variant)
                n7327 = Bundle By Name(cluster=w15586, "command"="MEAS.AllRelaysOFF") -> (w15594:T9)
                n7328 = Bundle By Name(cluster=w15586, "command"="MEAS.mux10-1", "data"=w15584) -> (w15577:T9)
                n7329 = Bundle By Name(cluster=w15586, "command"="MEAS.demux1-10", "data"=w15580) -> (w15578:T9)
                n7330 = Bundle By Name(cluster=w15586, "command"="MEAS.eMIC", "data"=w15595) -> (w15579:T9)
                n7331 = Build Array(w15594, w15577, w15578, w15579) -> (w15572:T9[])
                n7332 = To Variant(anything=w15576) -> (Variant=w15575:variant)
                n7333 = To Variant(anything=w15576) -> (Variant=w15574:variant)
                n7334 = Bundle By Name(cluster=w15573, "command"="MEAS.requestAC", "data"=w15575) -> (w15592:T9)
                n7335 = Bundle By Name(cluster=w15573, "command"="Apps.WaitForEvent", "data"=w15574) -> (w15588:T9)
                n7336 = Bundle By Name(cluster=w15573, "command"="Apps.UI Update 1") -> (w15589:T9)
                n7337 = Bundle By Name(cluster=w15573, "command"="WaitFor") -> (w15571:T9)
                n7338 = Build Array (concatenate)(w15572, w15571, w15592, w15588, w15589) -> (w15587:T9[])
              }
              frame True {
                w15602 = T9 {"command"="", "data"=variant} ("element")
                w15624 = T9 {"command"="", "data"=variant} ("element")
                n7339 = To Variant(anything=T3."mux10_1_channel10" ("mux10_1(x6)_encode")) -> (Variant=w15631:variant)
                n7340 = To Variant(anything=T2."mux6_1_channel4_3" ("mux6_1(3wires)_encode")) -> (Variant=w15629:variant)
                n7341 = To Variant(anything=T4."demux1_10_channel10" ("demux1_10(x6)_encode")) -> (Variant=w15625:variant)
                n7342 = To Variant(anything=bool[] [FALSE, FALSE, FALSE, TRUE, FALSE, FALSE]) -> (Variant=w15621:variant)
                n7343 = Bundle By Name(cluster=w15624, "command"="MEAS.AllRelaysOFF") -> (w15620:T9)
                n7344 = Bundle By Name(cluster=w15624, "command"="MEAS.mux10-1", "data"=w15631) -> (w15619:T9)
                n7345 = Bundle By Name(cluster=w15624, "command"="MEAS.mux6_1", "data"=w15629) -> (w15618:T9)
                n7346 = Bundle By Name(cluster=w15624, "command"="MEAS.demux1-10", "data"=w15625) -> (w15617:T9)
                n7347 = Bundle By Name(cluster=w15624, "command"="MEAS.eMIC", "data"=w15621) -> (w15616:T9)
                n7348 = Build Array(w15620, w15619, w15618, w15617, w15616) -> (w15601:T9[])
                n7349 = To Variant(anything=w15606) -> (Variant=w15604:variant)
                n7350 = To Variant(anything=w15606) -> (Variant=w15603:variant)
                n7351 = Bundle By Name(cluster=w15602, "command"="WaitFor") -> (w15600:T9)
                n7352 = Bundle By Name(cluster=w15602, "command"="MEAS.DMM dual read") -> (w15613:T9)
                n7353 = Bundle By Name(cluster=w15602, "command"="MEAS.requestAC", "data"=w15604) -> (w15612:T9)
                n7354 = Bundle By Name(cluster=w15602, "command"="Apps.WaitForEvent", "data"=w15603) -> (w15607:T9)
                n7355 = Bundle By Name(cluster=w15602, "command"="Apps.UI Update 1") -> (w15608:T9)
                n7356 = Build Array (concatenate)(w15601, w15600, w15613, w15612, w15607, w15608) -> (w15605:T9[])
              }
            }
          }
          frame True {
            n7357 = Bundle By Name(cluster=T9 {"command"="", "data"=variant} ("element"), "command"="Apps.UI Update 1") -> (w15635:T9)
            n7358 = Build Array(w15635) -> (w15634:T9[])
          }
        }
        n7359 = for {
          tunnel: w15550 -> [w15645] mode=indexing
          tunnel: w15558 -> [w15646]
          tunnel: [w15642] -> w15560 mode=indexing
          n7360 = Unbundle By Name(w15645) -> ("command"=w15644:string, "data"=w15643:variant)
          n7361 = call "App enquece.vi"("command data"=w15643, "command"=w15644, "queue in"=w15646) -> ("error out"=w15642:errorcluster)  [unwired: 7 in, 1 out]
        }
        n7362 = Merge Errors(w15561, w15560) -> (w15559:errorcluster)
      }
      frame "Test DRV 59A" {
        w15650 = 59 ("DUT index(0-59)")
        n7363 = disable-structure shown="LOGGING==TRUE" {
          disable-tunnel: w15655 -> [w15738 _]
          frame condition #0 (active) {
            n7364 = Empty String/Path?(string/path=w15738) -> (empty?=w15740:bool)
            n7365 = Select(t="Quece timeout", s=w15740, f=w15738) -> (s? t:f=w15737:string)
            n7366 = call "string log (SubVI).vi"("state Name"=w15737) -> ()  [unwired: 9 in, 2 out]
          }
          frame condition #1 {
          }
        }
        n7367 = Flush Queue(queue=w15656) -> (queue out=w15657:refnum<queue>)  [unwired: 1 in, 2 out]
        n7368 = Decrement(x=w15650) -> (x-1=w15654:i32)
        n7369 = Index Array(array=w15651, index=w15654) -> (element=w15652:refnum<vi>)
        n7370 = call "FGV DRV stand.vi"() -> ("Sub-Test.DCV"=w15647:bool)  [unwired: 10 in, 1 out]
        n7371 = call "FGV Driver Data.vi"("DUT index(1-60)"=w15650) -> ("DUT SC"=w15648:bool)  [unwired: 7 in, 3 out]
        n7372 = property class="ColBox"(reference=w15652, "Value"=u32 10000536 ("DRV 1")) -> ()  [unwired: 1 in, 2 out]
        n7373 = case shown="False" w15648 {
          tunnel: w15650 -> [w15668 _]
          tunnel: [w15667 w15733] -> w15649
          tunnel: w15647 -> [w15666 _]
          frame False {
            n7374 = case shown="True" w15666 {
              tunnel: w15668 -> [w15675 w15705]
              tunnel: [w15686 w15704] -> w15667
              frame False {
                w15672 = T9 {"command"="", "data"=variant} ("element")
                w15685 = T9 {"command"="", "data"=variant} ("element")
                n7375 = To Variant(anything=T3."mux10_1_channel10" ("mux10_1(x6)_encode")) -> (Variant=w15683:variant)
                n7376 = To Variant(anything=T4."demux1_10_channel10" ("demux1_10(x6)_encode")) -> (Variant=w15679:variant)
                n7377 = To Variant(anything=bool[] [FALSE, FALSE, FALSE, FALSE, TRUE, FALSE]) -> (Variant=w15694:variant)
                n7378 = Bundle By Name(cluster=w15685, "command"="MEAS.AllRelaysOFF") -> (w15693:T9)
                n7379 = Bundle By Name(cluster=w15685, "command"="MEAS.mux10-1", "data"=w15683) -> (w15676:T9)
                n7380 = Bundle By Name(cluster=w15685, "command"="MEAS.demux1-10", "data"=w15679) -> (w15677:T9)
                n7381 = Bundle By Name(cluster=w15685, "command"="MEAS.eMIC", "data"=w15694) -> (w15678:T9)
                n7382 = Build Array(w15693, w15676, w15677, w15678) -> (w15671:T9[])
                n7383 = To Variant(anything=w15675) -> (Variant=w15674:variant)
                n7384 = To Variant(anything=w15675) -> (Variant=w15673:variant)
                n7385 = Bundle By Name(cluster=w15672, "command"="MEAS.requestAC", "data"=w15674) -> (w15691:T9)
                n7386 = Bundle By Name(cluster=w15672, "command"="Apps.WaitForEvent", "data"=w15673) -> (w15687:T9)
                n7387 = Bundle By Name(cluster=w15672, "command"="Apps.UI Update 1") -> (w15688:T9)
                n7388 = Bundle By Name(cluster=w15672, "command"="WaitFor") -> (w15670:T9)
                n7389 = Build Array (concatenate)(w15671, w15670, w15691, w15687, w15688) -> (w15686:T9[])
              }
              frame True {
                w15701 = T9 {"command"="", "data"=variant} ("element")
                w15723 = T9 {"command"="", "data"=variant} ("element")
                n7390 = To Variant(anything=T3."mux10_1_channel10" ("mux10_1(x6)_encode")) -> (Variant=w15730:variant)
                n7391 = To Variant(anything=T2."mux6_1_channel5_3" ("mux6_1(3wires)_encode")) -> (Variant=w15728:variant)
                n7392 = To Variant(anything=T4."demux1_10_channel10" ("demux1_10(x6)_encode")) -> (Variant=w15724:variant)
                n7393 = To Variant(anything=bool[] [FALSE, FALSE, FALSE, FALSE, TRUE, FALSE]) -> (Variant=w15720:variant)
                n7394 = Bundle By Name(cluster=w15723, "command"="MEAS.AllRelaysOFF") -> (w15719:T9)
                n7395 = Bundle By Name(cluster=w15723, "command"="MEAS.mux10-1", "data"=w15730) -> (w15718:T9)
                n7396 = Bundle By Name(cluster=w15723, "command"="MEAS.mux6_1", "data"=w15728) -> (w15717:T9)
                n7397 = Bundle By Name(cluster=w15723, "command"="MEAS.demux1-10", "data"=w15724) -> (w15716:T9)
                n7398 = Bundle By Name(cluster=w15723, "command"="MEAS.eMIC", "data"=w15720) -> (w15715:T9)
                n7399 = Build Array(w15719, w15718, w15717, w15716, w15715) -> (w15700:T9[])
                n7400 = To Variant(anything=w15705) -> (Variant=w15703:variant)
                n7401 = To Variant(anything=w15705) -> (Variant=w15702:variant)
                n7402 = Bundle By Name(cluster=w15701, "command"="WaitFor") -> (w15699:T9)
                n7403 = Bundle By Name(cluster=w15701, "command"="MEAS.DMM dual read") -> (w15712:T9)
                n7404 = Bundle By Name(cluster=w15701, "command"="MEAS.requestAC", "data"=w15703) -> (w15711:T9)
                n7405 = Bundle By Name(cluster=w15701, "command"="Apps.WaitForEvent", "data"=w15702) -> (w15706:T9)
                n7406 = Bundle By Name(cluster=w15701, "command"="Apps.UI Update 1") -> (w15707:T9)
                n7407 = Build Array (concatenate)(w15700, w15699, w15712, w15711, w15706, w15707) -> (w15704:T9[])
              }
            }
          }
          frame True {
            n7408 = Bundle By Name(cluster=T9 {"command"="", "data"=variant} ("element"), "command"="Apps.UI Update 1") -> (w15734:T9)
            n7409 = Build Array(w15734) -> (w15733:T9[])
          }
        }
        n7410 = for {
          tunnel: w15649 -> [w15744] mode=indexing
          tunnel: w15657 -> [w15745]
          tunnel: [w15741] -> w15659 mode=indexing
          n7411 = Unbundle By Name(w15744) -> ("command"=w15743:string, "data"=w15742:variant)
          n7412 = call "App enquece.vi"("command data"=w15742, "command"=w15743, "queue in"=w15745) -> ("error out"=w15741:errorcluster)  [unwired: 7 in, 1 out]
        }
        n7413 = Merge Errors(w15660, w15659) -> (w15658:errorcluster)
      }
      frame "Test DRV 60A" {
        w15749 = 60 ("DUT index(0-59)")
        n7414 = disable-structure shown="LOGGING==TRUE" {
          disable-tunnel: w15754 -> [w15837 _]
          frame condition #0 (active) {
            n7415 = Empty String/Path?(string/path=w15837) -> (empty?=w15839:bool)
            n7416 = Select(t="Quece timeout", s=w15839, f=w15837) -> (s? t:f=w15836:string)
            n7417 = call "string log (SubVI).vi"("state Name"=w15836) -> ()  [unwired: 9 in, 2 out]
          }
          frame condition #1 {
          }
        }
        n7418 = Flush Queue(queue=w15755) -> (queue out=w15756:refnum<queue>)  [unwired: 1 in, 2 out]
        n7419 = Decrement(x=w15749) -> (x-1=w15753:i32)
        n7420 = Index Array(array=w15750, index=w15753) -> (element=w15751:refnum<vi>)
        n7421 = call "FGV DRV stand.vi"() -> ("Sub-Test.DCV"=w15746:bool)  [unwired: 10 in, 1 out]
        n7422 = call "FGV Driver Data.vi"("DUT index(1-60)"=w15749) -> ("DUT SC"=w15747:bool)  [unwired: 7 in, 3 out]
        n7423 = property class="ColBox"(reference=w15751, "Value"=u32 10000536 ("DRV 1")) -> ()  [unwired: 1 in, 2 out]
        n7424 = case shown="False" w15747 {
          tunnel: w15749 -> [w15767 _]
          tunnel: [w15766 w15832] -> w15748
          tunnel: w15746 -> [w15765 _]
          frame False {
            n7425 = case shown="False" w15765 {
              tunnel: w15767 -> [w15774 w15804]
              tunnel: [w15785 w15803] -> w15766
              frame False {
                w15771 = T9 {"command"="", "data"=variant} ("element")
                w15784 = T9 {"command"="", "data"=variant} ("element")
                n7426 = To Variant(anything=T3."mux10_1_channel10" ("mux10_1(x6)_encode")) -> (Variant=w15782:variant)
